vi "StackerSetpointIndex.vi"(8 "StackerCurrent":dbl format="%#_13g", 9 "Joystick Input":dbl format="%#_13g", 10 "On Bert?":bool=TRUE, 11 "StackerState":T1) -> (1 "Lock Setpoint as Current Height":bool, 2 "Travel Direction Up":bool, 3 "Setpoint":dbl)   [LabVIEW 2014]
uses:
  Typedefs/StackerStates.ctl
panel:
  in  "Ernie Stacker LUT":dbl[](array[numeric])=[0.0, 14.2, 14.2, 4.0, 0.4, 0.229, 4.0, 4.0]
  in  "Bert Stacker LUT":dbl[](array[numeric])=[0.0, 14.2, 14.2, 4.3, 0.5, 0.0, 5.0, 5.0]
  # "All of our stacker cals as recommended by Palardy, Eric do not fear I pledge to comment heavily on my \nLabview LUTs just like I do my C code LUTs in Vex."
  # "Manual"
  # "Manual"
  # "Hold 4"
  # "Hold 4"
  # "Hold 5"
  # "Hold 5"
  # "Hold 6"
  # "Hold 6"
  # "Get Tote"
  # "Get Tote"
  # "Drop Stack"
  # "Drop Stack"
  # "Hover Height"
  # "Hover Height"
  # "Hover for 5"
  # "Hover for 5"
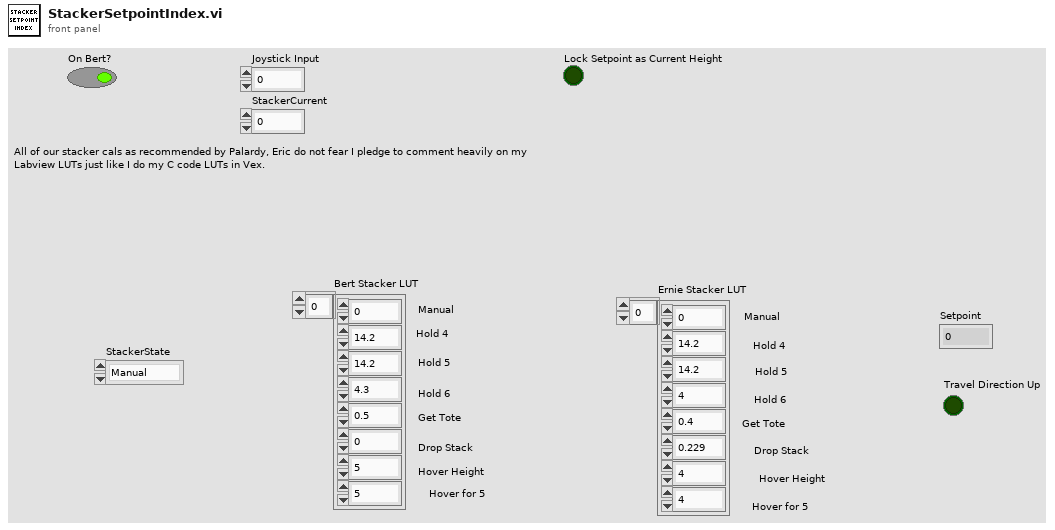
[diagram p1: front panel]
types:
  T1 = typedef "StackerStates.ctl" = enum16{"Manual ", "Hold", "Hold5", "Hold6", "GetTote", "DropStack", "Hover", "Hover5", "Wait for Up", "DecideHold", "DownTimerPeriod", "Prep Intake for Drop", "Check Arm before 5", "Make Arm ready for 5", "Check Arm before 6", "Make Arm ready for 6", "Delay for 5", "Delay for 6"}
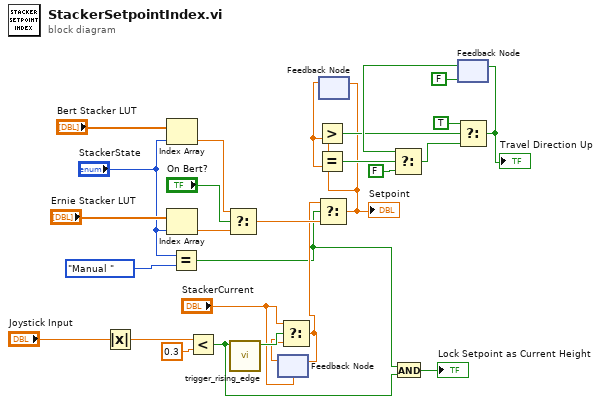
[diagram p0: block diagram]
diagram:
  n1 = Absolute Value(x="Joystick Input") -> (abs(x)=w12:dbl)
  n2 = Index Array(array="Bert Stacker LUT", index="StackerState") -> (element=w16:dbl)
  n3 = Index Array(array="Ernie Stacker LUT", index="StackerState") -> (element=w17:dbl)
  n4 = Equal?(x="StackerState", y=StackerStates."Manual ") -> (x = y?=w1:bool)
  n5 = Less?(x=w12, y=0.3) -> (x < y?=w2:bool)
  n6 = Select(t=w16, s="On Bert?", f=w17) -> (s? t:f=w9:dbl)
  n7 = call "trigger_rising_edge.vi"("input"=w2) -> ("rising"=w7:bool)  [unwired: 10 in]
  n8 = feedback #1("StackerCurrent") -> (w6:dbl)
  n9 = Select(t="StackerCurrent", s=w7, f=w6) -> (s? t:f=w4:dbl)
  n10 = feedback-in #1(w4) -> ()
  n11 = Select(t=w4, s=w1, f=w9) -> (s? t:f=w8:dbl)
  "Setpoint" <- w8
  n12 = feedback-in #2(w8) -> ()
  n13 = feedback #2() -> (w27:dbl)  [unwired: 1 in]
  n14 = Greater?(x=w8, y=w27) -> (0:w21:bool)
  n15 = Equal?(x=w8, y=w27) -> (x = y?=w24:bool)
  n16 = And(x=w1, y=w2) -> (x .and. y?=→"Lock Setpoint as Current Height":bool)
  n17 = feedback #3(FALSE) -> (w25:bool)
  n18 = Select(t=w25, s=w24, f=FALSE) -> (s? t:f=w23:bool)
  n19 = Select(t=TRUE, s=w21, f=w23) -> (s? t:f=w22:bool)
  "Travel Direction Up" <- w22
  n20 = feedback-in #3(w22) -> ()
